vi "performaction.vi"(11 "command line arguments":T1) -> (0 "error out":errorcluster)   [LabVIEW 2013]
uses:
  executables/arguments.ctl
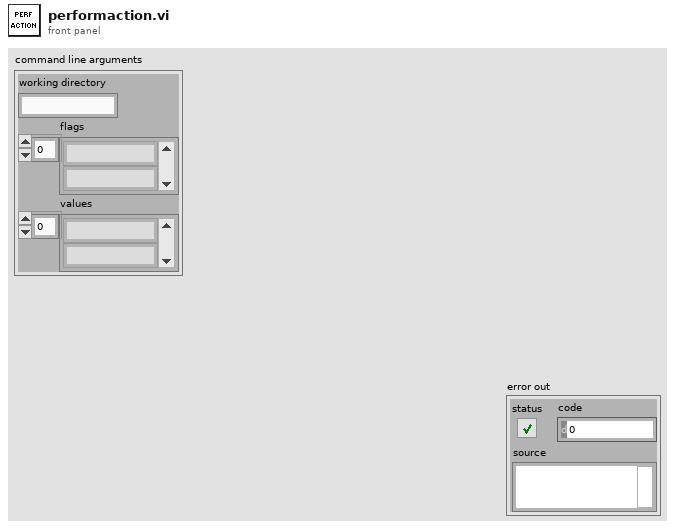
[diagram p1: front panel]
types:
  T1 = typedef "arguments.ctl" = cluster{"working directory":string, "flags":string[], "values":string[]}
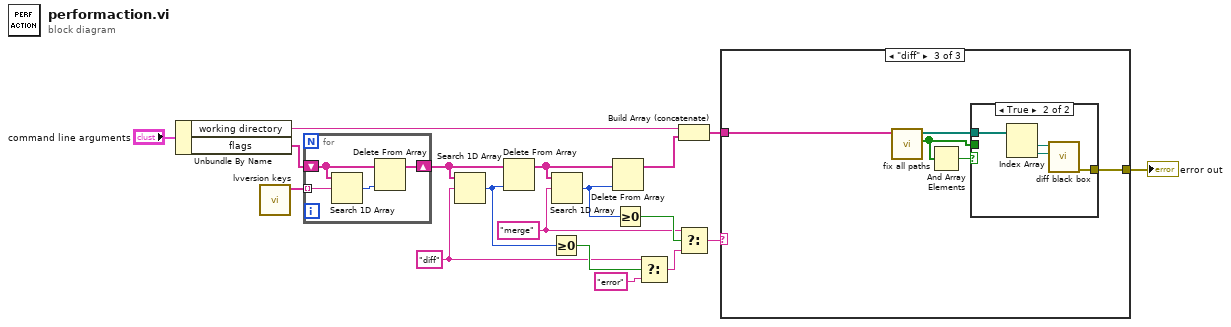
[diagram p0: block diagram]
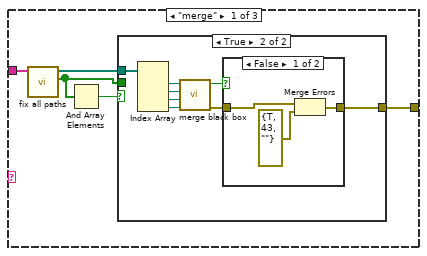
[diagram p2: hidden frame]
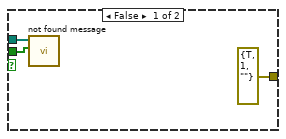
[diagram p3: hidden frame]
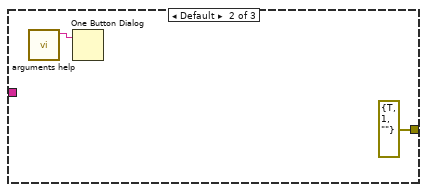
[diagram p5: hidden frame]
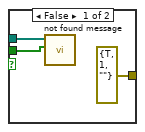
[diagram p6: hidden frame]
diagram:
  w5 = "merge" ("element")
  w4 = "diff" ("element")
  n1 = Unbundle By Name("command line arguments") -> ("working directory"=w16:string, "flags"=w15:string[])
  n2 = call "lvversion keys.vi"() -> ("lv version keys"=w14:string[])  [unwired: 11 in]
  n3 = for {
    shift-right: [w20] -> w13
    shift-left: w15 -> [w21]
    tunnel: w14 -> [w22] mode=indexing
    n4 = Search 1D Array(1D array=w21, element=w22) -> (index of element=w19:i32)  [unwired: 1 in]
    n5 = Delete From Array(array=w21, index=w19) -> (array with subset deleted=w20:string[])  [unwired: 1 in, 1 out]
  }
  n6 = Search 1D Array(1D array=w13, element=w4) -> (index of element=w9:i32)  [unwired: 1 in]
  n7 = Delete From Array(array=w13, index=w9) -> (array with subset deleted=w12:string[])  [unwired: 1 in, 1 out]
  n8 = Greater Or Equal To 0?(x=w9) -> (x >= 0?=w7:bool)
  n9 = Search 1D Array(1D array=w12, element=w5) -> (index of element=w8:i32)  [unwired: 1 in]
  n10 = Delete From Array(array=w12, index=w8) -> (array with subset deleted=w11:string[])  [unwired: 1 in, 1 out]
  n11 = Greater Or Equal To 0?(x=w8) -> (x >= 0?=w6:bool)
  n12 = Select(t=w4, s=w7, f="error" ("element")) -> (s? t:f=w3:string)
  n13 = Build Array (concatenate)(w16, w11) -> (w10:string[])
  n14 = Select(t=w5, s=w6, f=w3) -> (s? t:f=w1:string)
  n15 = case shown="\"diff\"" w1 {
    tunnel: w10 -> [w27 _ w46]
    tunnel: [w23 errorcluster {"status"=TRUE, "code"=1, "source"=""} ("error out") w45] -> w18
    frame "merge" {
      n16 = call "fix all paths.vi"("args"=w27) -> ("found"=w24:bool[], "paths out"=w25:path[])  [unwired: 9 in]
      n17 = And Array Elements(Boolean array=w24) -> (logical AND=w26:bool)
      n18 = case shown="True" w26 {
        tunnel: w25 -> [w30 w38]
        tunnel: w24 -> [w29 _]
        tunnel: [errorcluster {"status"=TRUE, "code"=1, "source"=""} ("error out") w32] -> w23
        frame False {
          n19 = call "not found message.vi"("found"=w29, "paths in"=w30) -> ()  [unwired: 10 in]
        }
        frame True {
          n20 = Index Array(array=w38) -> (element #1=w36:path, element #2=w35:path, element #3=w37:path, element #4=w34:path)  [unwired: 4 in]
          n21 = call "merge black box.vi"("merge"=w34, "yours"=w37, "their"=w35, "base"=w36) -> ("error out"=w31:errorcluster, "Saved?"=w33:bool)  [unwired: 6 in]
          n22 = case shown="False" w33 {
            tunnel: [w40 w42] -> w32
            tunnel: w31 -> [w41 w42]
            frame False {
              n23 = Merge Errors(w41, errorcluster {"status"=TRUE, "code"=43, "source"=""} ("error in")) -> (w40:errorcluster)
            }
            frame True {
            }
          }
        }
      }
    }
    frame Default {
      n24 = call "arguments help.vi"() -> ("args help"=w43:string)  [unwired: 11 in]
      n25 = One Button Dialog(message=w43) -> ()  [unwired: 1 in, 1 out]
    }
    frame "diff" {
      n26 = call "fix all paths.vi"("args"=w46) -> ("found"=w47:bool[], "paths out"=w48:path[])  [unwired: 9 in]
      n27 = And Array Elements(Boolean array=w47) -> (logical AND=w49:bool)
      n28 = case shown="True" w49 {
        tunnel: w48 -> [w52 w56]
        tunnel: w47 -> [w51 _]
        tunnel: [errorcluster {"status"=TRUE, "code"=1, "source"=""} ("error out") w53] -> w45
        frame False {
          n29 = call "not found message.vi"("found"=w51, "paths in"=w52) -> ()  [unwired: 10 in]
        }
        frame True {
          n30 = Index Array(array=w56) -> (element #1=w55:path, element #2=w54:path)  [unwired: 2 in]
          n31 = call "diff black box.vi"("VI2 Absolute"=w54, "VI1 Absolute"=w55) -> ("error out"=w53:errorcluster)  [unwired: 9 in]
        }
      }
    }
  }
  "error out" <- w18
